vi "[PC]SendCMD.vi"(9 "volume":dbl format="%#_g ml", 10 "temp":dbl, 11 "State Rqst":T1) -> ()   [LabVIEW 2018]
uses:
  TypeDef/ControllerState.ctl
  TypeDef/CMD Cluster.ctl
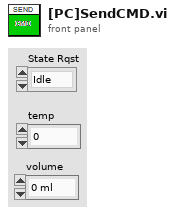
[diagram p1: front panel]
types:
  T1 = typedef "ControllerState.ctl" = enum16{"Idle", "Vorheizen", "Brühen", "Emergency-Stop"}
  T2 = typedef "CMD Cluster.ctl" = cluster{"timestamp":u32, "State Rqst":T1, "target-temp":dbl, "target-volume":dbl}
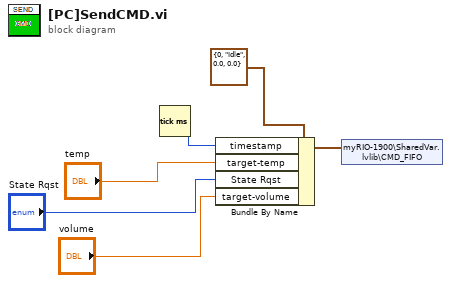
[diagram p0: block diagram]
diagram:
  n1 = Tick Count (ms)() -> (millisecond timer value=w3:u32)
  n2 = Bundle By Name(cluster=T2 {"timestamp"=0, "State Rqst"=enum."Idle", "target-temp"=0.0, "target-volume"=0.0} ("CMD_FIFO"), "timestamp"=w3, "target-temp"="temp", "State Rqst"="State Rqst", "target-volume"="volume") -> (w6:T2)
  n3 = shared-variable "myRIO-1900\\SharedVar.lvlib\\CMD_FIFO"(w6) -> ()  [unwired: 1 in, 1 out]
